vi "Clamp MAX_Main Function.vi"(5 "Refnum in":T3, 6 "ROI":T4, 8 "error in (no error)":errorcluster, 9 "Clamp Settings in":T8, 10 "Curve Extraction Settings in":T5, 11 "Overlay Settings":T6) -> (0 "error out":errorcluster, 1 "Clamp Points":T2, 2 "Clamp Results":T7, 3 "Refnum out":T3)   [LabVIEW 2019]
uses:
  <vilib>/vision/Image Controls.llb/IMAQ Image.ctl
  <vilib>/vision/NI_Vision_Development_Module.lvlib
panel:
  out "Coordinate System (duplicate)":T1 {"Measurement System"."Axis Reference" items=["Direct", "Indirect"]; "Measurement System"."Angle (deg)" format="%.2f"; "Measurement System"."Origin"."Y" format="%.2f"; "Measurement System"."Origin"."X" format="%.2f"; "Reference System"."Axis Reference" items=["Direct", "Indirect"]; "Reference System"."Angle (deg)" format="%.2f"; "Reference System"."Origin"."Y" format="%.2f"; "Reference System"."Origin"."X" format="%.2f"}
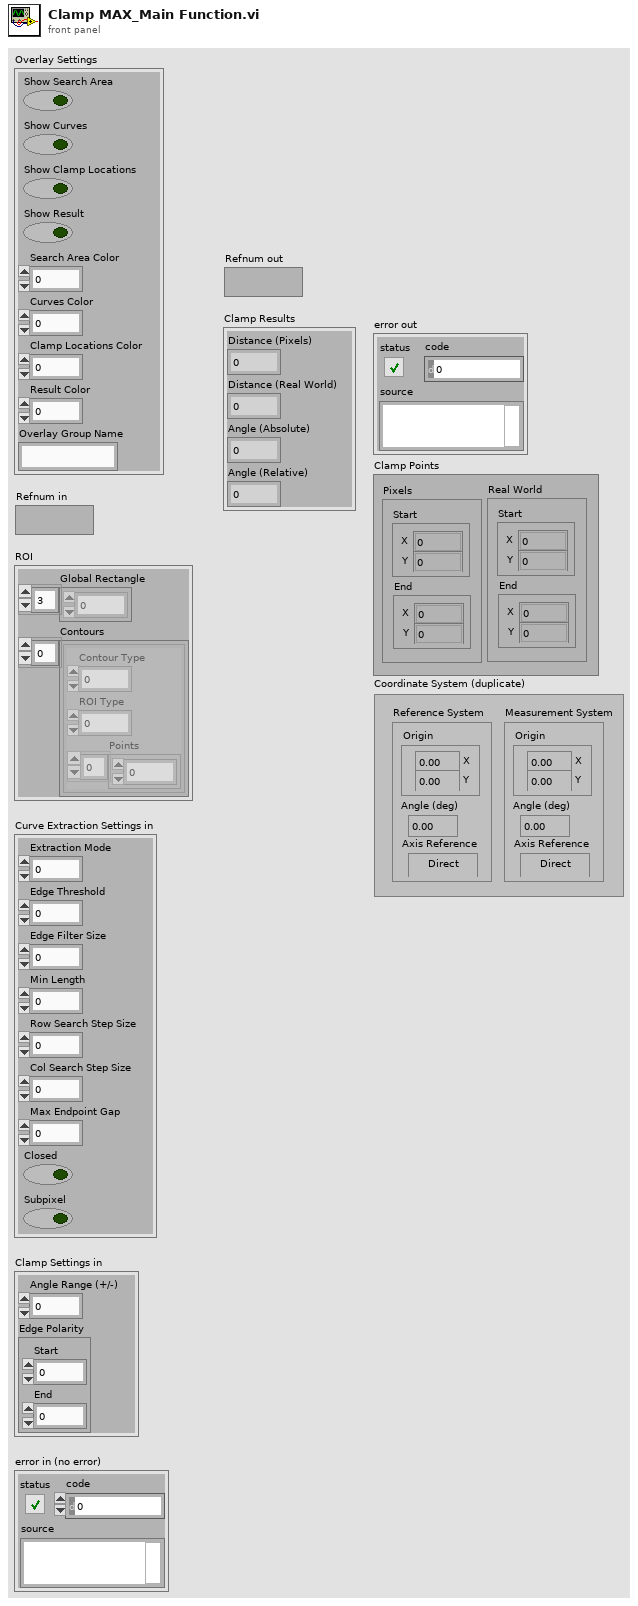
[diagram p1: front panel]
types:
  T1 = typedef "IMAQ Coordinate System" = cluster{"Reference System":cluster{"Origin":cluster{"X":sgl, "Y":sgl}, "Angle (deg)":sgl, "Axis Reference":u32}, "Measurement System":cluster{"Origin":cluster{"X":sgl, "Y":sgl}, "Angle (deg)":sgl, "Axis Reference":u32}}
  T2 = cluster{"Pixels ":cluster{"Start":cluster{"X":dbl, "Y":dbl}, "End":cluster{"X":dbl, "Y":dbl}}, "Real World":cluster{"Start":cluster{"X":dbl, "Y":dbl}, "End":cluster{"X":dbl, "Y":dbl}}}
  T3 = typedef "IMAQ Image.ctl" = refnum<image>
  T4 = cluster{"Global Rectangle":i32[], "Contours":cluster{"Contour Type":u32, "ROI Type":u32, "Points":i32[]}[]}
  T5 = cluster{"Extraction Mode":u32, "Edge Threshold":i32, "Edge Filter Size":u32, "Min Length":i32, "Row Search Step Size":i32, "Col Search Step Size":i32, "Max Endpoint Gap":i32, "Closed":bool, "Subpixel":bool}
  T6 = cluster{"Show Search Area":bool, "Show Curves":bool, "Show Clamp Locations":bool, "Show Result":bool, "Search Area Color":u32, "Curves Color":u32, "Clamp Locations Color":u32, "Result Color":u32, "Overlay Group Name":string}
  T7 = cluster{"Distance (Pixels)":dbl, "Distance (Real World)":dbl, "Angle (Absolute)":dbl, "Angle (Relative)":dbl}
  T8 = cluster{"Angle Range (+/-)":dbl, "Edge Polarity":cluster{"Start":u32, "End":u32}}
  T9 = typedef "ROI Descriptor" = cluster{"Global Rectangle":i32[], "Contours":cluster{"ID":enum32{"External", "Internal"}, "Type":u32, "Coordinates":i32[]}[]}
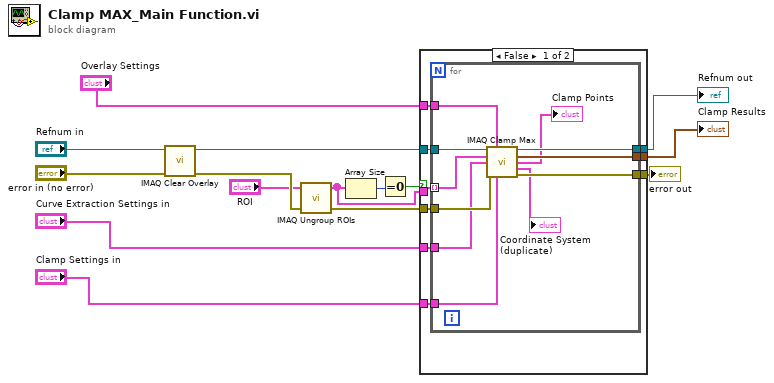
[diagram p0: block diagram]
diagram:
  n1 = call "IMAQ Clear Overlay"("error in (no error)"="error in (no error)", "Image"="Refnum in") -> ("error out"=w15:errorcluster, "Image Out"=w9:T3)  [unwired: 1 in, 7 out]
  n2 = call "IMAQ Ungroup ROIs"("error in (no error)"=w15, "ROI Descriptor"="ROI") -> ("error out"=w8:errorcluster, "ROI Descriptors out"=w1:T9[])  [unwired: 2 in]
  n3 = Array Size(array=w1) -> (size(s)=w3:i32)
  n4 = Equal To 0?(x=w3) -> (x = 0?=w2:bool)
  n5 = case shown="False" w2 {
    tunnel: "Clamp Settings in" -> [w24 _]
    tunnel: [w23 w37] -> w13
    tunnel: [w22 _] -> w12
    tunnel: "Overlay Settings" -> [w21 _]
    tunnel: "Curve Extraction Settings in" -> [w20 _]
    tunnel: w9 -> [w19 w37]
    tunnel: w8 -> [w18 w36]
    tunnel: [w17 w36] -> w5
    tunnel: w1 -> [w16 _]
    frame False {
      n6 = for {
        tunnel: w19 -> [w35]
        tunnel: w16 -> [w34] mode=indexing
        tunnel: w18 -> [w33]
        tunnel: w20 -> [w28]
        tunnel: w24 -> [w27]
        tunnel: w21 -> [w32]
        tunnel: [w31] -> w23
        tunnel: [w30] -> w22
        tunnel: [w29] -> w17
        n7 = call "IMAQ Clamp Max"("Source Image"=w35, "Overlay Settings"=w32, "ROI Descriptor"=w34, "Curve Extraction Settings"=w28, "error in (no error)"=w33, "Clamp Settings"=w27) -> ("Image Out"=w31:T3, "Clamp Results"=w30:T7, "Clamp Points"=→"Clamp Points":T2, "Coordinate System (duplicate)"=→"Coordinate System (duplicate)":T1, "error out"=w29:errorcluster)  [unwired: 1 in, 4 out]
      }
    }
    frame True {
    }
  }
  "Refnum out" <- w13
  "Clamp Results" <- w12
  "error out" <- w5
